vi "Read XML file to string array.vi"(8 "error in (no error)":errorcluster, 11 "path to XML document":path) -> (0 "error out":errorcluster, 3 "Array":string[][][](array[string]))   [LabVIEW 2020, in "XML Handler.lvclass"]
uses:
  XML Handler.lvclass
  <vilib>/xml/Load XML File.vi
  <vilib>/xml/Close Reference(NdList).vi
  <vilib>/xml/Close Reference(Node).vi
  <resource>/objmgr/DOMUserDefRef.rc
  <vilib>/xml/NI_XML.lvlib
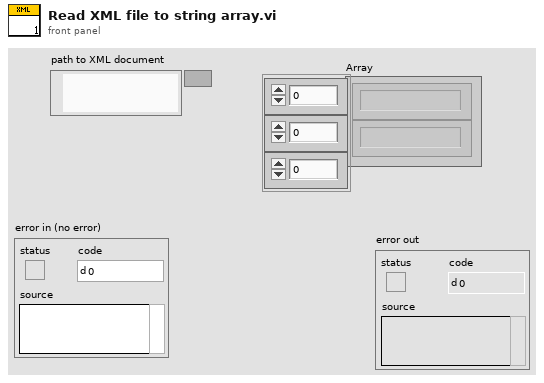
[diagram p1: front panel]
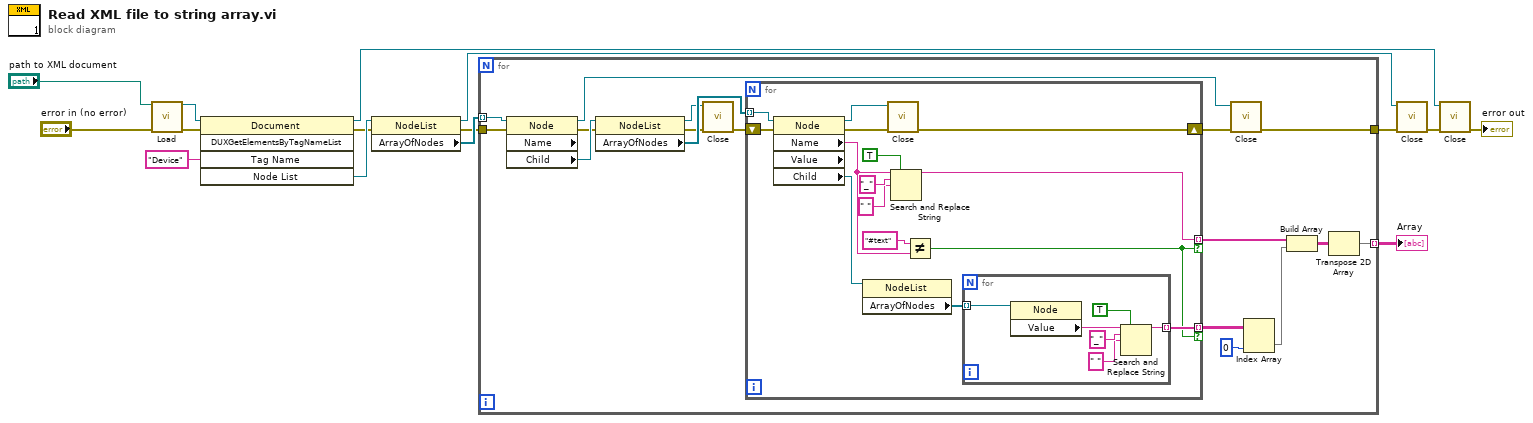
[diagram p0: block diagram]
diagram:
  n1 = call-poly <vilib>:"Load.vi"("path to XML document"="path to XML document", "error in (no error)"="error in (no error)") -> ("DOM document out"=w7:refnum<k20>, "error out"=w4:errorcluster)  [unwired: 11 in, 1 out]
  n2 = invoke class="Document" method="DUXGetElementsByTagNameList"(reference=w7, error in=w4, "Tag Name"="Device") -> (reference out=w14:refnum<k20>, error out=w3:errorcluster, "Node List"=w9:refnum<k20>)  [unwired: 2 in, 2 out]
  n3 = property class="NodeList"(reference=w9, error in=w3) -> (reference out=w11:refnum<k20>, error out=w2:errorcluster, "ArrayOfNodes"=w10:refnum<k20>[])
  n4 = for {
    tunnel: w10 -> [w32] mode=indexing
    tunnel: [w30] -> w12
    tunnel: [w22] -> w15 mode=indexing
    tunnel: w2 -> [w20]
    n5 = property class="Node" props=["Name", "Child"](reference=w32, error in=w20) -> (reference out=w31:refnum<k20>, error out=w19:errorcluster, "Child"=w29:refnum<k20>)  [unwired: 1 out]
    n6 = property class="NodeList"(reference=w29, error in=w19) -> (reference out=w27:refnum<k20>, error out=w18:errorcluster, "ArrayOfNodes"=w28:refnum<k20>[])
    n7 = call-poly <vilib>:"Close.vi"("error in (no error)"=w18, "node list"=w27) -> ("error out"=w17:errorcluster)  [unwired: 7 in]
    n8 = for {
      tunnel: w28 -> [w47] mode=indexing
      tunnel: [w39] -> w24 mode=indexing if=w41
      tunnel: [w43] -> w26 mode=indexing if=w41
      shift-right: [w33] -> w16
      shift-left: w17 -> [w35]
      n9 = property class="Node" props=["Name", "Value", "Child"](reference=w47, error in=w35) -> (reference out=w46:refnum<k20>, error out=w34:errorcluster, "Name"=w40:string, "Child"=w45:refnum<k20>)  [unwired: 1 out]
      n10 = property class="NodeList"(reference=w45) -> ("ArrayOfNodes"=w44:refnum<k20>[])  [unwired: 1 in, 2 out]
      n11 = call-poly <vilib>:"Close.vi"("error in (no error)"=w34, "node"=w46) -> ("error out"=w33:errorcluster)  [unwired: 7 in]
      n12 = Search and Replace String(replace all?=TRUE ("replace all? (F)"), input string=w40, search string="_", replace string=" " ("replace string (\"\")")) -> (result string=w39:string)  [unwired: 4 in, 3 out]
      n13 = Not Equal?(x="#text", y=w40) -> (x != y?=w41:bool)
      n14 = for {
        tunnel: w44 -> [w53] mode=indexing
        tunnel: [w48] -> w43 mode=indexing
        n15 = property class="Node"(reference=w53) -> ("Value"=w49:string)  [unwired: 1 in, 2 out]
        n16 = Search and Replace String(replace all?=TRUE ("replace all? (F)"), input string=w49, search string="_", replace string=" " ("replace string (\"\")")) -> (result string=w48:string)  [unwired: 4 in, 3 out]
      }
    }
    n17 = call-poly <vilib>:"Close.vi"("error in (no error)"=w16, "node"=w31) -> ("error out"=w30:errorcluster)  [unwired: 7 in]
    n18 = Index Array(array=w26, index (col)=0 ("disabled index (col)")) -> (element=w21:string[])  [unwired: 1 in]
    n19 = Build Array(w24, w21) -> (w23:string[][])
    n20 = Transpose 2D Array(2D array=w23) -> (transposed array=w22:string[][])
  }
  "Array" <- w15
  n21 = call-poly <vilib>:"Close.vi"("error in (no error)"=w12, "node list"=w11) -> ("error out"=w13:errorcluster)  [unwired: 7 in]
  n22 = call-poly <vilib>:"Close.vi"("error in (no error)"=w13, "node"=w14) -> ("error out"=→"error out":errorcluster)  [unwired: 7 in]
